vi "_Create (Protected).vi"(8 "error in (no error)":errorcluster, 11 "MockListImp in":refnum<class "ListImp_RefSpy.lvclass">) -> (0 "error out":errorcluster, 3 "MockListImp out":refnum<class "ListImp_RefSpy.lvclass">)   [LabVIEW 2013, in "ListImp_RefSpy.lvclass"]
doc: "This method is invoked when the List:Create method is called. Child implementations should override this method to initialize or obtain any runtime resource needed. \n\nChild classes do not need to wrap the code in an error case."
uses:
  ListImp_RefSpy.lvclass
  RefnumGlobal.vi
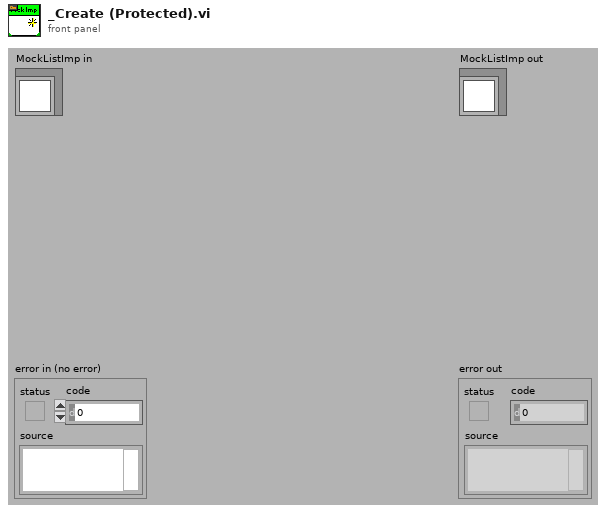
[diagram p1: front panel]
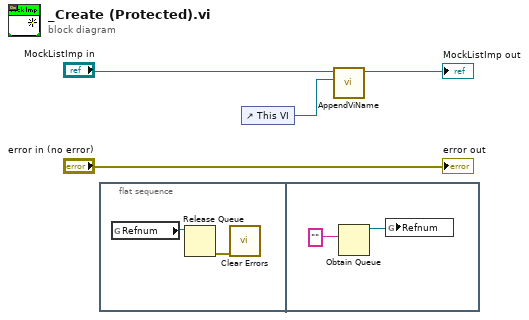
[diagram p0: block diagram]
diagram:
  n1 = flat-sequence {
    frame #0 {
      n2 = global read "RefnumGlobal.vi" "Refnum"() -> (w6:refnum<queue>)
      n3 = Release Queue(queue=w6) -> (error out=w5:errorcluster)  [unwired: 2 in, 2 out]
      n4 = call <vilib>:"Clear Errors.vi"("error in (no error)"=w5) -> ()  [unwired: 5 in, 2 out]
    }
    frame #1 {
      n5 = Obtain Queue(element data type="") -> (queue out=w8:refnum<queue>)  [unwired: 4 in, 2 out]
      n6 = global write "RefnumGlobal.vi" "Refnum"(w8) -> ()
    }
  }
  n7 = control-ref of="This VI"() -> (w1:refnum<vi>)
  n8 = call "AppendViName.vi"("VI Refnum"=w1, "MockListImp in"="MockListImp in") -> ("MockListImp out"=→"MockListImp out":refnum<class "ListImp_RefSpy.lvclass">)  [unwired: 8 in, 1 out]
  "error out" <- "error in (no error)"
